vi "GUIAS CURVAS EM FUNÇÃO DO RAIO-7.vi"() -> ()   [LabVIEW 2014]
uses:
  <vilib>/Instr/_visa.llb/VISA Configure Serial Port (Instr).vi
  <userlib>/Newport ESP301/Newport ESP301.lvlib
panel:
  out "Numeric Control":i32
  in  "Velocity":dbl=3.0
  out "Raio":dbl
  out "PROGRESSÃO":i32
  in  "Raios":dbl[](array[numeric])=[40.0, 60.0, 80.0, 100.0, 120.0, 140.0, 180.0]
  in  "N_Guias":dbl=7.0
  in  "Iniciar":bool
  in  "L":dbl=10.0 format="%.1f"
  in  "In.Curva":dbl=2.0
  out "d (um)":dbl
  in  "Distância (um)":dbl=50.0
  in  "Stop Button":bool
  # "Inicio curva"
  # "Tam.amostra (mm)"
  # "Núm.guias"
  # "Raio (mm)"
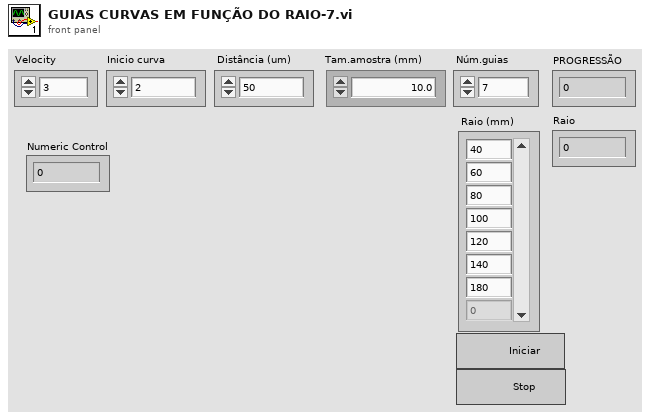
[diagram p1: front panel]
types:
  T1 = cluster{"Axis1 moving":bool, "Axis2 moving":bool, "Axis3 moving":bool, "Axis4 moving":bool, "Motor Power of at least one axis":bool, "Reserved":bool, "Reserved":bool, "Reserved":bool, "Axis5 moving 2":bool, "Axis6 moving 2":bool, "Reserved":bool, "Reserved":bool, "Motor Power of at least one axis":bool, "Reserved":bool, "Reserved":bool, "Reserved":bool}
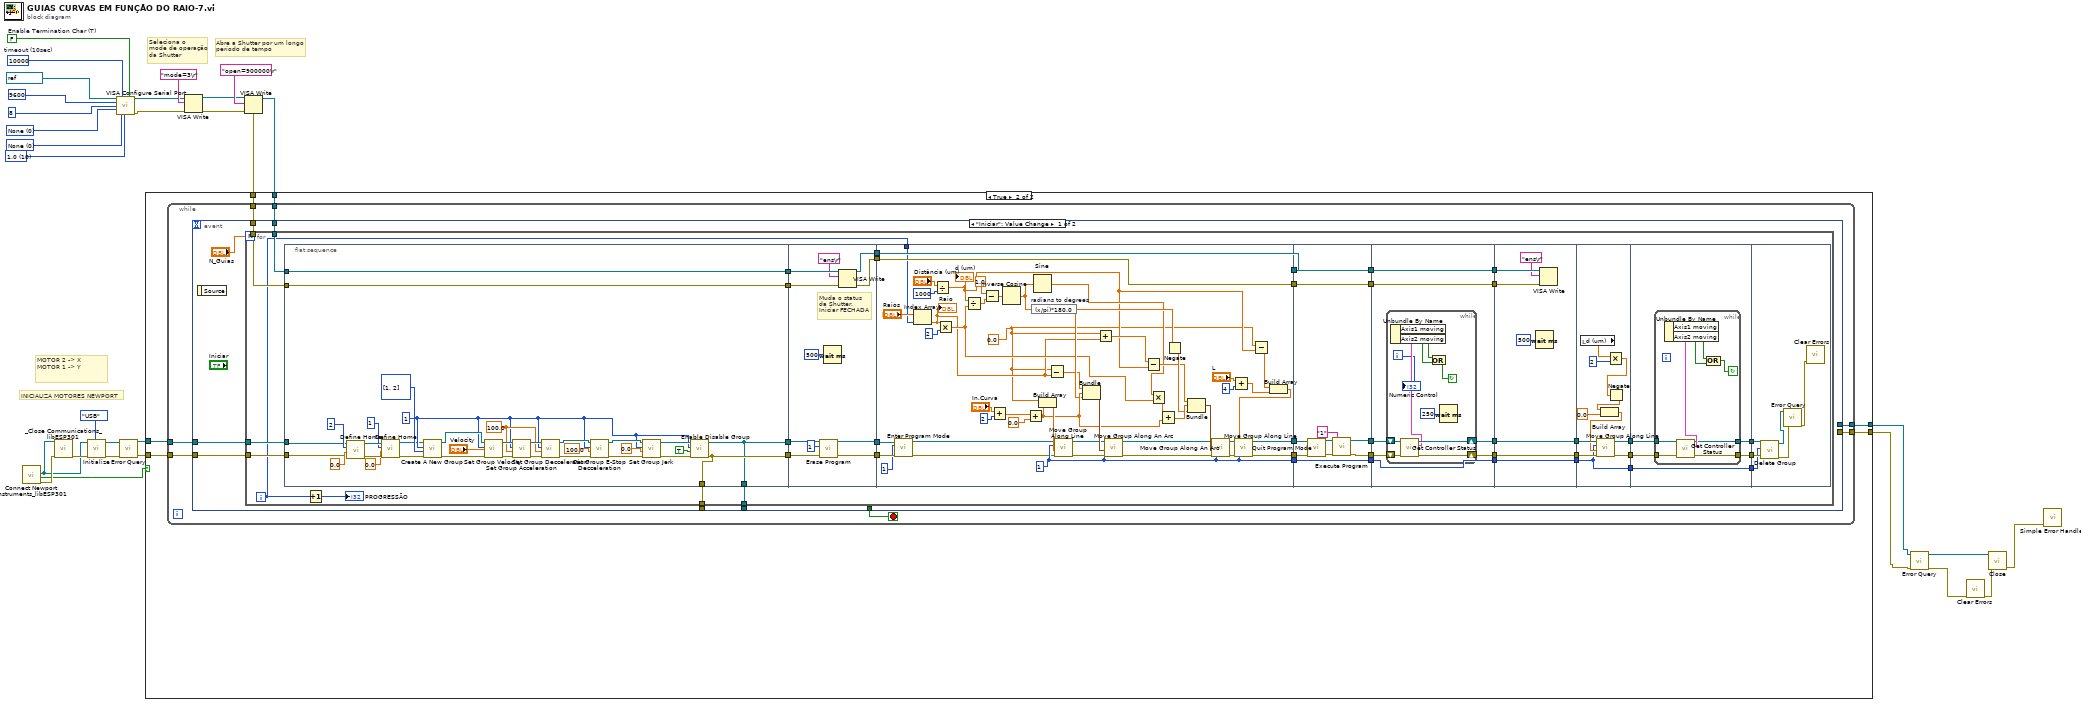
[diagram p0: block diagram]
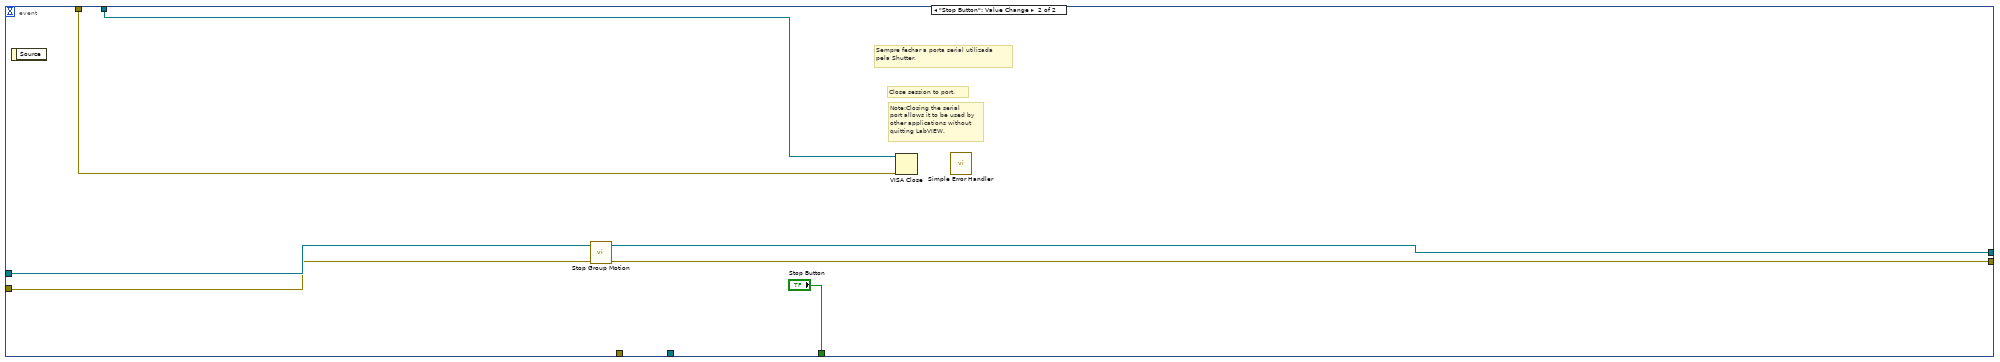
[diagram p3: hidden frame]
diagram:
  w12 = u16 0 items=["None", "Odd", "Even", "Mark", "Space"] ("parity")
  w15 = u16 10 items=["1.0"=10, "1.5"=15, "2.0"=20] ("stop bits")
  w16 = u16 0 items=["None"=0, "XON/XOFF"=1, "RTS/CTS"=2, "DTR/DSR"=4] ("flow control")
  w14 = FALSE  # Enable Termination Char (T)
  w13 = u32 10000  # timeout (10sec)
  # "Abre a Shutter por um longo\nperíodo de tempo"
  # "Seleciona o \nmode de operação\nda Shutter"
  # "MOTOR 2 -> X\nMOTOR 1 -> Y"
  # "INICIALIZA MOTORES NEWPORT"
  n1 = call <userlib>:"Connect Newport Instruments_libESP301.vi"() -> ("error (duplicate)"=w29:errorcluster, "Connected"=w21:bool, "VISA resource name (duplicate)"=w28:refnum<visa-resource-name>)  [unwired: 7 in, 2 out]
  n2 = call <userlib>:"_Close Communications_libESP301.vi"("Instrument Channel"=w28, "error in (no error)"=w29) -> ("error out"=w31:errorcluster)  [unwired: 13 in]
  n3 = call <userlib>:"Initialize.vi"("VISA resource name"=w28, "error in (no error)"=w31, "Serial Link (RS232)"=enum16{"RS232", "USB"}."USB") -> ("VISA resource name out"=w27:refnum<visa-resource-name>, "error out"=w26:errorcluster)  [unwired: 6 in]
  n4 = call-poly "VISA Configure Serial Port"("VISA resource name"=refnum<visa-resource-name> "COM6", "timeout (10sec)"=w13, "Enable Termination\nChar (T)"=w14, "baud rate (9600)"=u32 9600 ("baud rate"), "data bits (8)"=u16 8 ("data bits"), "parity (0:none)"=w12, "stop bits (10: 1 bit)"=w15, "flow control (0:none)"=w16) -> ("VISA resource name out"=w8:refnum<visa-resource-name>, "error out"=w7:errorcluster)  [unwired: 6 in]
  n5 = call <userlib>:"Error Query.vi"("error in (no error)"=w26, "VISA resource name"=w27) -> ("error out"=w18:errorcluster, "VISA resource name out"=w19:refnum<visa-resource-name>)  [unwired: 2 in, 2 out]
  n6 = VISA Write(VISA resource name=w8, write buffer="mode=3\r", error in (no error)=w7) -> (VISA resource name out=w5:refnum<visa-resource-name>, error out=w4:errorcluster)  [unwired: 1 out]
  n7 = VISA Write(VISA resource name=w5, write buffer="open=900000\r", error in (no error)=w4) -> (VISA resource name out=w22:refnum<visa-resource-name>, error out=w20:errorcluster)  [unwired: 1 out]
  n8 = case shown="True" w21 {
    tunnel: w19 -> [w33 w36]
    tunnel: w18 -> [w32 w37]
    tunnel: w22 -> [_ w39]
    tunnel: w20 -> [_ w38]
    tunnel: [w33 w35] -> w3
    tunnel: [w32 w34] -> w2
    frame False {
    }
    frame True {
      n9 = while {
        tunnel: w37 -> [w46]
        tunnel: w36 -> [w45]
        tunnel: w39 -> [w43]
        tunnel: w38 -> [w42]
        tunnel: [w41] -> w35
        tunnel: [w40] -> w34
        stop <- w44 stop-if-true
        n10 = event shown="[0] \"Iniciar\": Value Change" {
          selector: _ -> [_ _]
          dyn-events: _ -> [_ _]
          timeout: _ -> [_ _]
          tunnel: w46 -> [w53 w255]
          tunnel: w45 -> [w52 w256]
          tunnel: [_ "Stop Button"] -> w44
          tunnel: w43 -> [w50 w257]
          tunnel: w42 -> [w49 w254]
          tunnel: [w48 _] -> _
          tunnel: [w47 _] -> _
          tunnel: [_ w253] -> w41
          tunnel: [_ w252] -> w40
          event "Iniciar": Value Change {
            n11 = event-data() -> ()  [unwired: 1 in, 1 out]
            n12 = for {
              N: "N_Guias" -> [_]
              tunnel: w53 -> [w91]
              tunnel: w52 -> [w90]
              tunnel: w50 -> [w88]
              tunnel: w49 -> [w75]
              tunnel: [w65] -> w48
              tunnel: [w64] -> w47
              i -> [w74]
              n13 = flat-sequence {
                tunnel: w75 -> [w125]
                tunnel: w88 -> [w126]
                tunnel: w90 -> [w97]
                tunnel: w91 -> [w96]
                tunnel: [w95] -> w73
                tunnel: [w94] -> w72
                tunnel: [w126] -> w71
                tunnel: [w125] -> w70
                tunnel: [w95] -> w65
                tunnel: [w94] -> w64
                tunnel: [w128] -> w93
                tunnel: [w129] -> w92
                tunnel: [w135] -> w81
                tunnel: [w134] -> w79
                tunnel: w73 -> [w130]
                tunnel: w72 -> [w131]
                tunnel: w71 -> [w136]
                tunnel: w70 -> [w133]
                tunnel: w93 -> [w142]
                tunnel: w92 -> [w141]
                tunnel: w74 -> [w160]
                tunnel: [w149] -> w63
                tunnel: [w164] -> w61
                tunnel: [w163] -> w59
                tunnel: w81 -> [w161]
                tunnel: [w162] -> w57
                tunnel: w79 -> [w162]
                tunnel: [w161] -> w55
                tunnel: w63 -> [w197]
                tunnel: [w197] -> w62
                tunnel: w61 -> [w193]
                tunnel: [w189] -> w60
                tunnel: w59 -> [w194]
                tunnel: [w190] -> w58
                tunnel: w57 -> [w196]
                tunnel: [w196] -> w56
                tunnel: w55 -> [w195]
                tunnel: [w195] -> w54
                tunnel: [w204] -> w86
                tunnel: w62 -> [w204]
                tunnel: w60 -> [w200]
                tunnel: [w198] -> w85
                tunnel: w58 -> [w201]
                tunnel: [w199] -> w83
                tunnel: [w203] -> w80
                tunnel: w56 -> [w203]
                tunnel: w54 -> [w202]
                tunnel: [w202] -> w78
                tunnel: [w221] -> w87
                tunnel: w86 -> [w221]
                tunnel: w85 -> [w220]
                tunnel: [w220] -> w84
                tunnel: w83 -> [w219]
                tunnel: [w219] -> w82
                tunnel: w80 -> [w218]
                tunnel: w78 -> [w217]
                tunnel: w87 -> [w222]
                tunnel: w84 -> [w232]
                tunnel: w82 -> [w231]
                tunnel: [w225] -> w77
                tunnel: [w224] -> w76
                tunnel: [w222] -> w66
                tunnel: w77 -> [w237]
                tunnel: w76 -> [w236]
                tunnel: [w235] -> w69
                tunnel: [w234] -> w68
                tunnel: [w233] -> w67
                tunnel: w66 -> [w233]
                tunnel: w69 -> [w251]
                tunnel: w68 -> [w250]
                tunnel: w67 -> [w249]
                frame #0 {
                  w106 = 1 ("Group #")
                  w116 = 100.0 ("Acceleration (0 units/s²)")
                  n14 = call <userlib>:"Define Home.vi"("error in (no error)"=w96, "Home Position (0 units)"=0.0, "Axis (1)"=2 ("y"), "VISA resource name"=w97) -> ("error out"=w104:errorcluster, "VISA resource name out"=w105:refnum<visa-resource-name>)  [unwired: 2 in]
                  n15 = call <userlib>:"Define Home.vi"("error in (no error)"=w104, "Home Position (0 units)"=0.0, "Axis (1)"=1, "VISA resource name"=w105) -> ("error out"=w98:errorcluster, "VISA resource name out"=w99:refnum<visa-resource-name>)  [unwired: 2 in]
                  n16 = call <userlib>:"Create A New Group.vi"("error in (no error)"=w98, "Axis Number"=i32[] [1, 2], "Group Number (1)"=w106, "VISA resource name"=w99) -> ("error out"=w122:errorcluster, "VISA resource name out"=w123:refnum<visa-resource-name>)  [unwired: 2 in]
                  n17 = call <userlib>:"Set Group Velocity.vi"("error in (no error)"=w122, "Velocity (units/s)"="Velocity", "Group Number (1)"=w106, "VISA resource name"=w123) -> ("error out"=w117:errorcluster, "VISA resource name out"=w120:refnum<visa-resource-name>)  [unwired: 2 in]
                  n18 = call <userlib>:"Set Group Acceleration.vi"("error in (no error)"=w117, "Acceleration (0 units/s²)"=w116, "Group Number (1)"=w106, "VISA resource name"=w120) -> ("error out"=w118:errorcluster, "VISA resource name out"=w119:refnum<visa-resource-name>)  [unwired: 2 in]
                  n19 = call <userlib>:"Set Group Decceleration.vi"("error in (no error)"=w118, "Decceleration (0 units/s²)"=w116, "Group Number (1)"=w106, "VISA resource name"=w119) -> ("error out"=w112:errorcluster, "VISA resource name out"=w115:refnum<visa-resource-name>)  [unwired: 2 in]
                  n20 = call <userlib>:"Set Group E-Stop Decceleration.vi"("error in (no error)"=w112, "E-Stop Decceleration (0 units/s²)"=100.0, "Group Number (1)"=w106, "VISA resource name"=w115) -> ("error out"=w111:errorcluster, "VISA resource name out"=w114:refnum<visa-resource-name>)  [unwired: 2 in]
                  n21 = call <userlib>:"Set Group Jerk.vi"("error in (no error)"=w111, "Vector Jerk (0 units/s^3)"=0.0, "Group Number (1)"=w106, "VISA resource name"=w114) -> ("error out"=w110:errorcluster, "VISA resource name out"=w113:refnum<visa-resource-name>)  [unwired: 2 in]
                  n22 = call <userlib>:"Enable Disable Group.vi"("error in (no error)"=w110, "Action (OFF)"=TRUE, "Group Number (1)"=w106, "VISA resource name"=w113) -> ("error out"=w95:errorcluster, "VISA resource name out"=w94:refnum<visa-resource-name>)  [unwired: 2 in]
                }
                frame #1 {
                  # "Muda o status\nda Shutter.\nIniciar FECHADA"
                  n23 = call <userlib>:"Erase Program.vi"("error in (no error)"=w130, "Program # (1)"=1, "VISA resource name"=w131) -> ("error out"=w128:errorcluster, "VISA resource name out"=w129:refnum<visa-resource-name>)  [unwired: 3 in]
                  n24 = Wait (ms)(milliseconds to wait=u32 500) -> ()  [unwired: 1 out]
                  n25 = VISA Write(VISA resource name=w136, write buffer="ens\r", error in (no error)=w133) -> (VISA resource name out=w135:refnum<visa-resource-name>, error out=w134:errorcluster)  [unwired: 1 out]
                }
                frame #2 {
                  w151 = 0.0 ("x")
                  w149 = 1 ("y")
                  n26 = call <userlib>:"Enter Program Mode.vi"("error in (no error)"=w142, "Program Number (1)"=1, "VISA resource name"=w141) -> ("error out"=w139:errorcluster, "VISA resource name out"=w140:refnum<visa-resource-name>)  [unwired: 3 in]
                  n27 = Index Array(array="Raios", index=w160) -> (element=w153:dbl)
                  "Raio" <- w153
                  n28 = Divide(x="Distância (um)", y=1000) -> (x/y=w152:dbl)
                  "d (um)" <- w152
                  n29 = Multiply(x=w153, y=2) -> (x*y=w155:dbl)
                  n30 = Divide(x=w152, y=w155) -> (x/y=w183:dbl)
                  n31 = Subtract(x=1.0, y=w183) -> (x-y=w181:dbl)
                  n32 = Add(x="In.Curva", y=2) -> (x+y=w173:dbl)
                  n33 = Inverse Cosine(1:w181) -> (0:w174:dbl)
                  n34 = Add(x=w173, y=0.0) -> (x+y=w171:dbl)
                  n35 = expression code="(x/pi)*180.0" "radians to degrees"(w174) -> (w167:dbl)
                  n36 = Sine(x=w174) -> (sin(x)=w154:dbl)
                  n37 = Build Array(w151, w171) -> (w178:dbl[])
                  n38 = Subtract(x=w151, y=w153) -> (x-y=w158:dbl)
                  n39 = call <userlib>:"Move Group Along Line.vi"("error in (no error)"=w139, "Position (0 units)"=w178, "Group Number (1)"=w149, "VISA resource name"=w140) -> ("error out"=w143:errorcluster, "VISA resource name out"=w144:refnum<visa-resource-name>)  [unwired: 2 in]
                  n40 = Bundle(w158, w171, w167) -> (w177:cluster{dbl, dbl, dbl})  [unwired: 1 in]
                  n41 = Add(x=w151, y=w153) -> (x+y=w157:dbl)
                  n42 = call <userlib>:"Move Group Along An Arc.vi"("error in (no error)"=w143, "Arc  Parameters"=w177, "Group Number (1)"=w149, "VISA resource name"=w144) -> ("error out"=w147:errorcluster, "VISA resource name out"=w148:refnum<visa-resource-name>)  [unwired: 2 in]
                  n43 = Subtract(x=w157, y=w152) -> (x-y=w156:dbl)
                  n44 = Multiply(x=w154, y=w155) -> (x*y=w172:dbl)
                  n45 = Add(x=w172, y=w171) -> (x+y=w170:dbl)
                  n46 = Negate(x=w167) -> (-x=w166:dbl)
                  n47 = Bundle(w156, w170, w166) -> (w187:cluster{dbl, dbl, dbl})  [unwired: 1 in]
                  n48 = call <userlib>:"Move Group Along An Arc.vi"("error in (no error)"=w147, "Arc  Parameters"=w187, "Group Number (1)"=w149, "VISA resource name"=w148) -> ("error out"=w145:errorcluster, "VISA resource name out"=w146:refnum<visa-resource-name>)  [unwired: 2 in]
                  n49 = Add(x="L", y=4) -> (x+y=w169:dbl)
                  n50 = Subtract(x=w151, y=w152) -> (x-y=w159:dbl)
                  n51 = Build Array(w159, w169) -> (w168:dbl[])
                  n52 = call <userlib>:"Move Group Along Line.vi"("error in (no error)"=w145, "Position (0 units)"=w168, "Group Number (1)"=w149, "VISA resource name"=w146) -> ("error out"=w164:errorcluster, "VISA resource name out"=w163:refnum<visa-resource-name>)  [unwired: 2 in]
                }
                frame #3 {
                  n53 = call <userlib>:"Quit Program Mode.vi"("error in (no error)"=w193, "VISA resource name"=w194) -> ("error out"=w191:errorcluster, "VISA resource name out"=w192:refnum<visa-resource-name>)  [unwired: 4 in]
                  n54 = call <userlib>:"Execute Program.vi"("error in (no error)"=w191, "Program Name"="1", "VISA resource name"=w192) -> ("error out"=w189:errorcluster, "VISA resource name out"=w190:refnum<visa-resource-name>)  [unwired: 3 in]
                }
                frame #4 {
                  n55 = while {
                    shift-right: [w212] -> w199
                    shift-left: w201 -> [w214]
                    shift-right: [w211] -> w198
                    shift-left: w200 -> [w213]
                    i -> [w206]
                    stop <- w207 continue-if-true
                    n56 = call <userlib>:"Get Controller Status.vi"("error in (no error)"=w213, "VISA resource name"=w214) -> ("error out"=w211:errorcluster, "Controller Status"=w210:T1, "VISA resource name out"=w212:refnum<visa-resource-name>)  [unwired: 2 in, 1 out]
                    n57 = Unbundle By Name(w210) -> ("Axis1 moving"=w209:bool, "Axis2 moving"=w208:bool)
                    n58 = Compound Arithmetic op=OR(w209, w208) -> (w207:bool)
                    n59 = Wait (ms)(milliseconds to wait=u32 250) -> ()  [unwired: 1 out]
                    "Numeric Control" <- w206
                  }
                }
                frame #5 {
                  n60 = Wait (ms)(milliseconds to wait=u32 500) -> ()  [unwired: 1 out]
                  n61 = VISA Write(VISA resource name=w217, write buffer="ens\r", error in (no error)=w218) -> ()  [unwired: 3 out]
                }
                frame #6 {
                  n62 = local read "d (um)"() -> (w228:dbl)
                  n63 = Multiply(x=w228, y=2) -> (x*y=w223:dbl)
                  n64 = Negate(x=w223) -> (-x=w226:dbl)
                  n65 = Build Array(w226, 0.0 ("element")) -> (w230:dbl[])
                  n66 = call <userlib>:"Move Group Along Line.vi"("error in (no error)"=w232, "Position (0 units)"=w230, "Group Number (1)"=w222, "VISA resource name"=w231) -> ("error out"=w224:errorcluster, "VISA resource name out"=w225:refnum<visa-resource-name>)  [unwired: 2 in]
                }
                frame #7 {
                  n67 = while {
                    tunnel: w237 -> [w241]
                    tunnel: w236 -> [w240]
                    tunnel: [w239] -> w235
                    tunnel: [w238] -> w234
                    stop <- w242 continue-if-true
                    n68 = call <userlib>:"Get Controller Status.vi"("error in (no error)"=w240, "VISA resource name"=w241) -> ("error out"=w238:errorcluster, "Controller Status"=w245:T1, "VISA resource name out"=w239:refnum<visa-resource-name>)  [unwired: 2 in, 1 out]
                    n69 = Unbundle By Name(w245) -> ("Axis1 moving"=w244:bool, "Axis2 moving"=w243:bool)
                    n70 = Compound Arithmetic op=OR(w244, w243) -> (w242:bool)
                  }
                }
                frame #8 {
                  n71 = call <userlib>:"Delete Group.vi"("error in (no error)"=w250, "Group Number (1)"=w249, "VISA resource name"=w251) -> ("error out"=w246:errorcluster, "VISA resource name out"=w247:refnum<visa-resource-name>)  [unwired: 3 in]
                  n72 = call <userlib>:"Error Query.vi"("error in (no error)"=w246, "VISA resource name"=w247) -> ("error out"=w248:errorcluster)  [unwired: 2 in, 3 out]
                  n73 = call <vilib>:"Clear Errors.vi"("error in (no error)"=w248) -> ()  [unwired: 5 in, 2 out]
                }
              }
              n74 = Increment(x=w74) -> (x+1=→"PROGRESSÃO":i32)
            }
          }
          event "Stop Button": Value Change {
            # "Sempre fechar a porta serial utilizada\npela Shutter."
            # "Note:Closing the serial port allows it to be used by other applications without\nquitting LabVIEW."
            # "Close session to port."
            n75 = event-data() -> ()  [unwired: 1 in, 1 out]
            n76 = call <userlib>:"Stop Group Motion.vi"("error in (no error)"=w255, "VISA resource name"=w256) -> ("error out"=w252:errorcluster, "VISA resource name out"=w253:refnum<visa-resource-name>)  [unwired: 4 in]
            n77 = VISA Close(VISA resource name=w257, error in (no error)=w254) -> ()  [unwired: 1 out]
            n78 = call <vilib>:"Simple Error Handler.vi"() -> ()  [unwired: 5 in, 5 out]
          }
        }
      }
    }
  }
  n79 = call <userlib>:"Error Query.vi"("error in (no error)"=w2, "VISA resource name"=w3) -> ("error out"=w23:errorcluster, "VISA resource name out"=w24:refnum<visa-resource-name>)  [unwired: 2 in, 2 out]
  n80 = call <vilib>:"Clear Errors.vi"("error in (no error)"=w23) -> ("error out"=w25:errorcluster)  [unwired: 5 in, 1 out]
  n81 = call <userlib>:"Close.vi"("error in (no error)"=w25, "VISA resource name"=w24) -> ("error out"=w1:errorcluster)  [unwired: 9 in]
  n82 = call <vilib>:"Simple Error Handler.vi"("error in (no error)"=w1) -> ()  [unwired: 4 in, 5 out]
